vi "DeviceOff.vi"(8 "error in (no error)":errorcluster, 11 "PacificPowerSource in":refnum<class "PacificPowerSource.lvclass">) -> (0 "error out":errorcluster, 3 "PacificPowerSource out":refnum<class "PacificPowerSource.lvclass">)   [LabVIEW 2018, in "AcPwrPlugins.lvlib" / "PacificPowerSource.lvclass"]
doc: "This VI sets the output to off by opening the output switch."
uses:
  PacificPowerSource.lvclass
  <instrlib>/Pacific Power UPC Series/Pacific Power UPC Series.lvlib
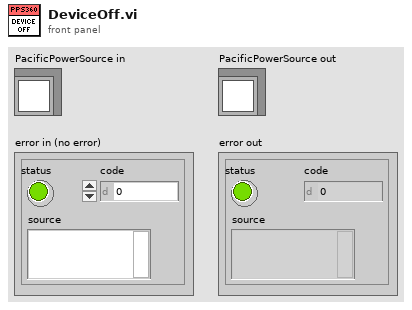
[diagram p1: front panel]
types:
  T1 = typedef "AcPwrPlugins.lvlib/PacificPowerSource.lvclass/Device(s)Settings.ctl" = cluster{"MeasName":string, "Modules":cluster{"Handle":string, "Connected":bool, "Clear Device (F)":bool, "btnIdQuery":bool, "btnReset":bool, "Program #":cluster{"Phase B (Degrees)":i32, "Waveform A (1: Sine)":i32, "Voltage Level (Va)":dbl, "Program Number (0)":i32, "Voltage Level (Vb) ":dbl, "Form (3: Three)":u16, "Coupling  (0: Direct)":u16, "Frequency (45Hz)":dbl, "Current Limit (40A)":dbl, "Phase C (Degrees)":i32, "Voltage Level (Vc)":dbl, "Waveform B (1: Sine)":i32, "Waveform C (1: Sine)":i32}[], "Impedance Parameters (off, 0.00)":cluster{"State":bool, "Impedance":dbl}, "Transient Execution (F)":bool, "OutputEnabled":bool, "Source Range":cluster{"Frequency Minimum (45 Hz)":dbl, "Frequency Maximum (1200 Hz)":dbl, "Voltage Maximum (V)":dbl, "Voltage Minimum (V)":dbl, "Range Control (0: Auto)":u16, "Initial Voltage (0V)":u16, "Frequency Range (600Hz)":u16}, "Port Type":enum16{"GPIB", "Serial"}}[]}
  T2 = typedef "AcPwrPlugins.lvlib/PacificPowerSource.lvclass/Measurements.ctl" = cluster{"Handle":string, "Name":string, "Enabled ":bool, "Measurement Value":dbl, "Channel Name":enum16{"A", "B", "C"}, "Measurement Type ":T3}[]
  T3 = typedef "AcPwrPlugins.lvlib/PacificPowerSource.lvclass/MeasurementType.ctl" = enum16{"Voltage RMS L-N", "Voltage RMS L-L", "Frequency", "Current RMS", "Current Peak", "Crest Factor", "Power Factor", "Power VA", "Real Power"}
  T4 = typedef "AcPwrPlugins.lvlib/PacificPowerSource.lvclass/Modules.ctl" = cluster{"Handle":string, "Connected":bool, "Clear Device (F)":bool, "btnIdQuery":bool, "btnReset":bool, "Program #":cluster{"Phase B (Degrees)":i32, "Waveform A (1: Sine)":i32, "Voltage Level (Va)":dbl, "Program Number (0)":i32, "Voltage Level (Vb) ":dbl, "Form (3: Three)":u16, "Coupling  (0: Direct)":u16, "Frequency (45Hz)":dbl, "Current Limit (40A)":dbl, "Phase C (Degrees)":i32, "Voltage Level (Vc)":dbl, "Waveform B (1: Sine)":i32, "Waveform C (1: Sine)":i32}[], "Impedance Parameters (off, 0.00)":cluster{"State":bool, "Impedance":dbl}, "Transient Execution (F)":bool, "OutputEnabled":bool, "Source Range":cluster{"Frequency Minimum (45 Hz)":dbl, "Frequency Maximum (1200 Hz)":dbl, "Voltage Maximum (V)":dbl, "Voltage Minimum (V)":dbl, "Range Control (0: Auto)":u16, "Initial Voltage (0V)":u16, "Frequency Range (600Hz)":u16}, "Port Type":enum16{"GPIB", "Serial"}}[]
  T5 = cluster{"Phase B (Degrees)":i32, "Waveform A (1: Sine)":i32, "Voltage Level (Va)":dbl, "Program Number (0)":i32, "Voltage Level (Vb) ":dbl, "Form (3: Three)":u16, "Coupling  (0: Direct)":u16, "Frequency (45Hz)":dbl, "Current Limit (40A)":dbl, "Phase C (Degrees)":i32, "Voltage Level (Vc)":dbl, "Waveform B (1: Sine)":i32, "Waveform C (1: Sine)":i32}[]
  T6 = cluster{"Phase B (Degrees)":i32, "Waveform A (1: Sine)":i32, "Voltage Level (Va)":dbl, "Program Number (0)":i32, "Voltage Level (Vb) ":dbl, "Form (3: Three)":u16, "Coupling  (0: Direct)":u16, "Frequency (45Hz)":dbl, "Current Limit (40A)":dbl, "Phase C (Degrees)":i32, "Voltage Level (Vc)":dbl, "Waveform B (1: Sine)":i32, "Waveform C (1: Sine)":i32}
  T7 = cluster{"Handle":string, "Connected":bool, "Clear Device (F)":bool, "btnIdQuery":bool, "btnReset":bool, "Program #":cluster{"Phase B (Degrees)":i32, "Waveform A (1: Sine)":i32, "Voltage Level (Va)":dbl, "Program Number (0)":i32, "Voltage Level (Vb) ":dbl, "Form (3: Three)":u16, "Coupling  (0: Direct)":u16, "Frequency (45Hz)":dbl, "Current Limit (40A)":dbl, "Phase C (Degrees)":i32, "Voltage Level (Vc)":dbl, "Waveform B (1: Sine)":i32, "Waveform C (1: Sine)":i32}[], "Impedance Parameters (off, 0.00)":cluster{"State":bool, "Impedance":dbl}, "Transient Execution (F)":bool, "OutputEnabled":bool, "Source Range":cluster{"Frequency Minimum (45 Hz)":dbl, "Frequency Maximum (1200 Hz)":dbl, "Voltage Maximum (V)":dbl, "Voltage Minimum (V)":dbl, "Range Control (0: Auto)":u16, "Initial Voltage (0V)":u16, "Frequency Range (600Hz)":u16}, "Port Type":enum16{"GPIB", "Serial"}}
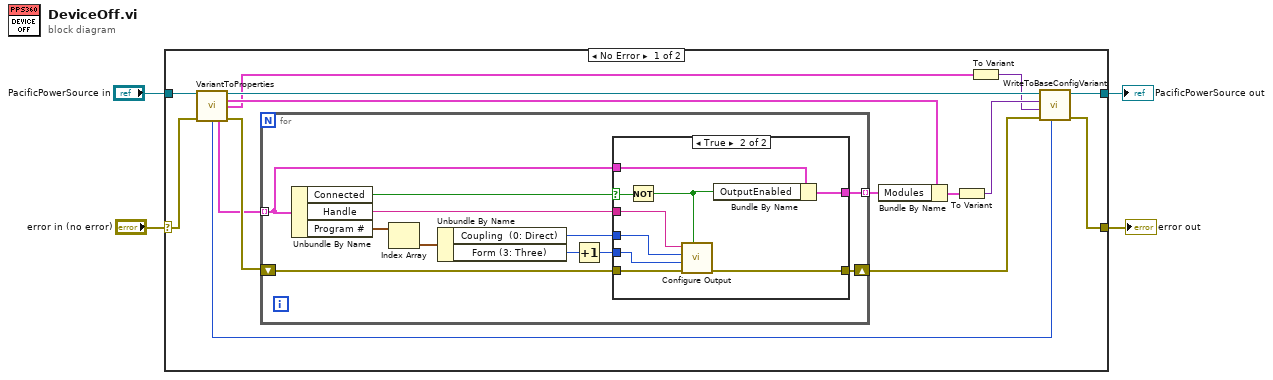
[diagram p0: block diagram]
diagram:
  n1 = case shown="No Error" "error in (no error)" {
    selector: "error in (no error)" -> [w17 w43]
    tunnel: [w8 w43] -> w1
    tunnel: [w10 w42] -> w2
    tunnel: "PacificPowerSource in" -> [w18 w42]
    frame No Error {
      n2 = call "VariantToProperties.vi"("PacificPowerSource in"=w18, "error in (no error)"=w17) -> ("PacificPowerSource out"=w9:refnum<class "PacificPowerSource.lvclass">, "Device(s)Settings"=w14:T1, "Measurements"=w5:T2, "Measurement Refresh Time (ms)"=w7:u32, "Modules"=w15:T4, "error out"=w16:errorcluster)  [unwired: 7 in, 1 out]
      n3 = for {
        tunnel: w15 -> [w26] mode=indexing
        shift-right: [w27] -> w13
        shift-left: w16 -> [w28]
        tunnel: [w25] -> w19 mode=indexing
        n4 = Unbundle By Name(w26) -> ("Connected"=w29:bool, "Handle"=w30:string, "Program #"=w22:T5)
        n5 = Index Array(array=w22) -> (element=w24:T6)  [unwired: 1 in]
        n6 = Unbundle By Name(w24) -> ("Coupling  (0: Direct)"=w21:u16, "Form (3: Three)"=w23:u16)
        n7 = Increment(x=w23) -> (x+1=w20:u16)
        n8 = case shown="True" w29 {
          selector: w29 -> [_ w39]
          tunnel: w28 -> [w32 w40]
          tunnel: [w32 w41] -> w27
          tunnel: w30 -> [_ w38]
          tunnel: w26 -> [w31 w37]
          tunnel: [w31 w35] -> w25
          tunnel: w21 -> [_ w34]
          tunnel: w20 -> [_ w33]
          frame False {
          }
          frame True {
            n9 = Not(x=w39) -> (.not. x?=w36:bool)
            n10 = call <instrlib>:"Configure Output.vi"("Enable Output (T: Enable)"=w36, "error in (no error)"=w40, "Form (3: Three)"=w33, "Coupling  (0: Direct)"=w34, "VISA resource name"=w38) -> ("error out"=w41:errorcluster)  [unwired: 5 in, 1 out]
            n11 = Bundle By Name(cluster=w37, "OutputEnabled"=w36) -> (w35:T7)
          }
        }
      }
      n12 = Bundle By Name(cluster=w14, "Modules"=w19) -> (w11:T1)
      n13 = To Variant(anything=w11) -> (Variant=w12:variant)
      n14 = To Variant(anything=w5) -> (Variant=w6:variant)
      n15 = call "WriteToBaseConfigVariant.vi"("Measurement Refresh Time (ms)"=w7, "error in (no error)"=w13, "Meas"=w6, "Config"=w12, "PacificPowerSource in"=w9) -> ("error out"=w8:errorcluster, "PacificPowerSource out"=w10:refnum<class "PacificPowerSource.lvclass">)  [unwired: 5 in]
    }
    frame Error {
    }
  }
  "error out" <- w1
  "PacificPowerSource out" <- w2
